vi "ofdm_subcarrier_partitioner.vi"(9 "message carrier":u32, 10 "FFT size":u32, 11 "received symbol":cdb[](array[numeric])) -> (0 "pilot subcarriers":cdb[](array[numeric]), 3 "message subcarriers":cdb[](array[numeric]))   [LabVIEW 2020]
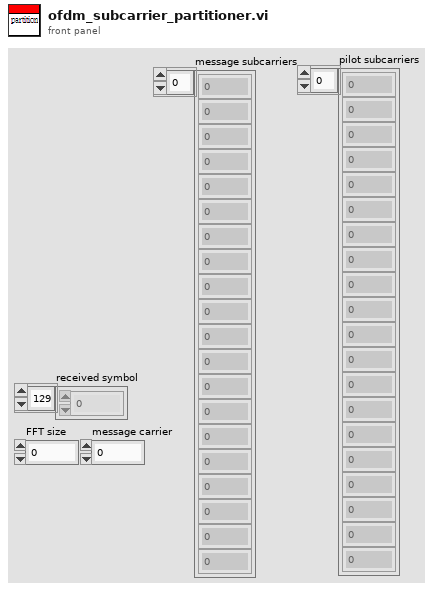
[diagram p1: front panel]
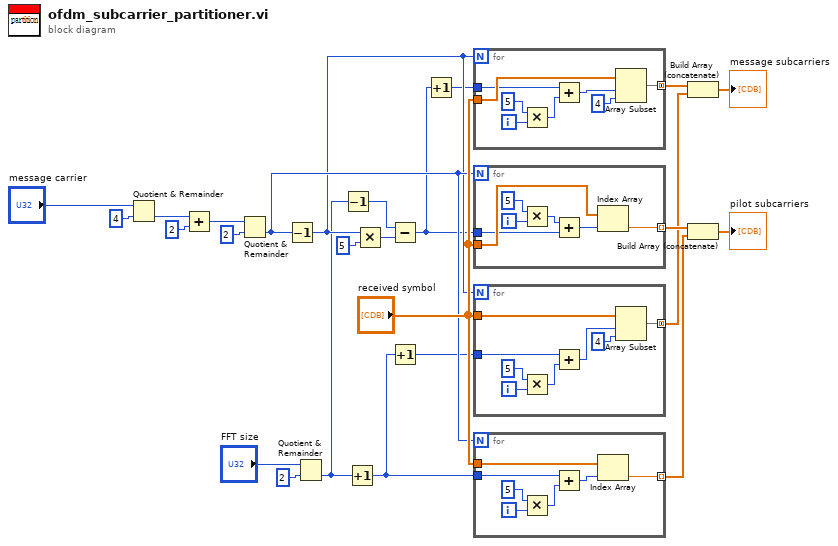
[diagram p0: block diagram]
diagram:
  n1 = Quotient & Remainder(x="message carrier", y=4) -> (floor(x/y)=w3:u32)  [unwired: 1 out]
  n2 = Add(x=w3, y=2) -> (x+y=w1:u32)
  n3 = Quotient & Remainder(x=w1, y=2) -> (floor(x/y)=w13:u32)  [unwired: 1 out]
  n4 = Decrement(x=w13) -> (x-1=w12:u32)
  n5 = Quotient & Remainder(x="FFT size", y=2) -> (floor(x/y)=w10:u32)  [unwired: 1 out]
  n6 = Decrement(x=w10) -> (x-1=w11:u32)
  n7 = Increment(x=w10) -> (x+1=w8:u32)
  n8 = Multiply(x=w12, y=5) -> (x*y=w20:u32)
  n9 = Subtract(x=w11, y=w20) -> (x-y=w6:u32)
  n10 = Increment(x=w8) -> (x+1=w9:u32)
  n11 = Increment(x=w6) -> (x+1=w7:u32)
  n12 = for {
    N: w12 -> [_]
    tunnel: "received symbol" -> [w31]
    tunnel: w7 -> [w28]
    tunnel: [w26] -> w16 mode=concatenating
    i -> [w32]
    n13 = Multiply(x=5, y=w32) -> (x*y=w29:i32)
    n14 = Add(x=w28, y=w29) -> (x+y=w30:u32)
    n15 = Array Subset(array=w31, index=w30, length=4) -> (w26:cdb[])
  }
  n16 = for {
    N: w13 -> [_]
    tunnel: "received symbol" -> [w40]
    tunnel: w6 -> [w38]
    tunnel: [w37] -> w19 mode=indexing
    i -> [w36]
    n17 = Multiply(x=5, y=w36) -> (x*y=w35:i32)
    n18 = Add(x=w35, y=w38) -> (x+y=w39:u32)
    n19 = Index Array(array=w40, index=w39) -> (element=w37:cdb)
  }
  n20 = for {
    N: w12 -> [_]
    tunnel: w9 -> [w46]
    tunnel: "received symbol" -> [w48]
    tunnel: [w45] -> w18 mode=concatenating
    i -> [w43]
    n21 = Multiply(x=5, y=w43) -> (x*y=w44:i32)
    n22 = Add(x=w46, y=w44) -> (x+y=w47:u32)
    n23 = Array Subset(array=w48, index=w47, length=4) -> (w45:cdb[])
  }
  n24 = for {
    N: w13 -> [_]
    tunnel: w8 -> [w54]
    tunnel: "received symbol" -> [w53]
    tunnel: [w49] -> w22 mode=indexing
    i -> [w52]
    n25 = Multiply(x=5, y=w52) -> (x*y=w51:i32)
    n26 = Add(x=w54, y=w51) -> (x+y=w55:u32)
    n27 = Index Array(array=w53, index=w55) -> (element=w49:cdb)
  }
  n28 = Build Array (concatenate)(w16, w18) -> (→"message subcarriers":cdb[])
  n29 = Build Array (concatenate)(w19, w22) -> (→"pilot subcarriers":cdb[])
